vi "new_nerualnetwork_test.vi"() -> ()   [LabVIEW 2014]
panel:
  out "Output Layer":dbl[](array[numeric])
  out "HiDen Layer":dbl[](array[numeric])
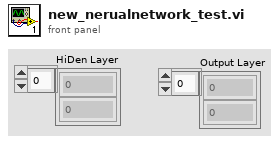
[diagram p1: front panel]
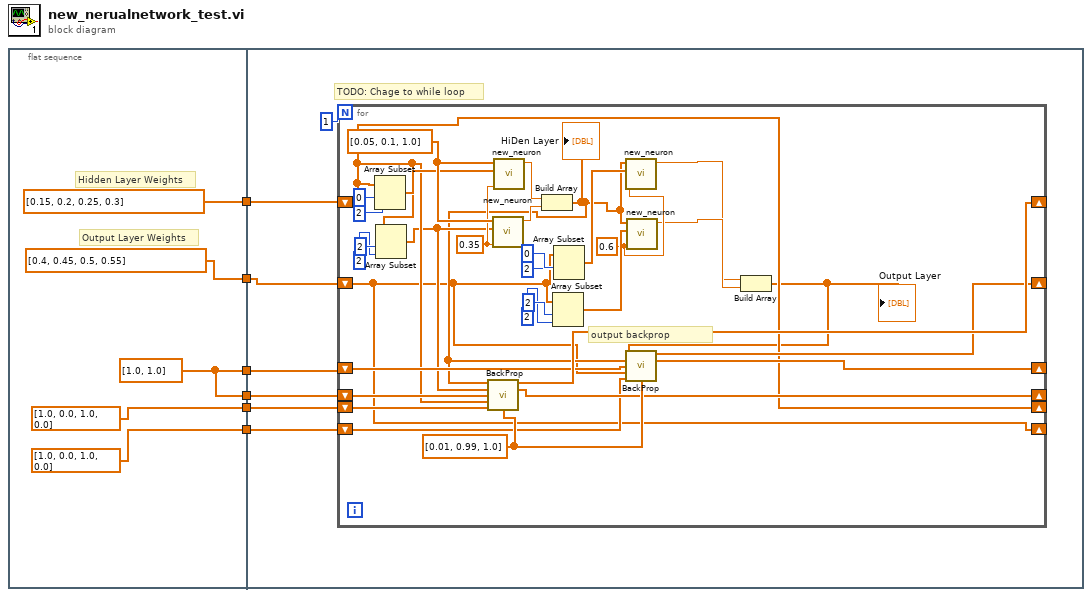
[diagram p0: block diagram]
diagram:
  n1 = flat-sequence {
    tunnel: [dbl[] [0.15, 0.2, 0.25, 0.3] ("Target")] -> w6
    tunnel: [dbl[] [0.4, 0.45, 0.5, 0.55] ("Target")] -> w5
    tunnel: [w9] -> w4
    tunnel: [w9] -> w3
    tunnel: [dbl[] [1.0, 0.0, 1.0, 0.0] ("PreviousWeights")] -> w2
    tunnel: [dbl[] [1.0, 0.0, 1.0, 0.0] ("PreviousWeights")] -> w1
    tunnel: w6 -> [w18]
    tunnel: w5 -> [w16]
    tunnel: w4 -> [w15]
    tunnel: w3 -> [w14]
    tunnel: w2 -> [w13]
    tunnel: w1 -> [w12]
    frame #0 {
      w9 = dbl[] [1.0, 1.0] ("dE_dNET")
      # "Output Layer Weights"
      # "Hidden Layer Weights"
    }
    frame #1 {
      # "TODO: Chage to while loop"
      n2 = for {
        N: 1 -> [_]
        shift-right: [w29] -> _
        shift-left: w16 -> [w19]
        shift-right: [w30] -> _
        shift-left: w18 -> [w24]
        shift-right: [w31] -> _
        shift-left: w15 -> [w26]
        shift-right: [w28] -> _
        shift-left: w14 -> [w27]
        shift-right: [w24] -> _
        shift-left: w13 -> [w25]
        shift-right: [w19] -> _
        shift-left: w12 -> [w23]
        w35 = 0.6 ("Offset")
        w36 = 0.35 ("Offset")
        w50 = dbl[] [0.05, 0.1, 1.0] ("Target")
        w32 = dbl[] [0.01, 0.99, 1.0] ("Target")
        # "output backprop"
        n3 = Array Subset(array=w24, index=0, length=2) -> (w45:dbl[])
        n4 = Array Subset(array=w24, index=2, length=2) -> (w22:dbl[])
        n5 = call "new_neuron.vi"("Offset"=w36, "Weights"=w22, "Inputs"=w50) -> ("Output"=w43:dbl)  [unwired: 8 in]
        n6 = call "new_neuron.vi"("Offset"=w36, "Weights"=w45, "Inputs"=w50) -> ("Output"=w44:dbl)  [unwired: 8 in]
        n7 = Build Array(w44, w43) -> (w21:dbl[])
        "HiDen Layer" <- w21
        n8 = call "BackProp.vi"("Current Layer"=w21, "Previous Layer"=w22, "NetError"=w27, "weights"=w24, "PreviousWeights"=w25, "Target"=w32) -> ("w+"=w30:dbl[], "dE_dNET"=w28:dbl[])  [unwired: 8 in]
        n9 = Array Subset(array=w19, index=2, length=2) -> (w38:dbl[])
        n10 = Array Subset(array=w19, index=0, length=2) -> (w37:dbl[])
        n11 = call "new_neuron.vi"("Offset"=w35, "Weights"=w37, "Inputs"=w21) -> ("Output"=w33:dbl)  [unwired: 8 in]
        n12 = call "new_neuron.vi"("Offset"=w35, "Weights"=w38, "Inputs"=w21) -> ("Output"=w34:dbl)  [unwired: 8 in]
        n13 = Build Array(w33, w34) -> (w20:dbl[])
        "Output Layer" <- w20
        n14 = call "BackProp.vi"("Current Layer"=w20, "Previous Layer"=w21, "NetError"=w26, "weights"=w19, "PreviousWeights"=w23, "Target"=w32) -> ("w+"=w29:dbl[], "dE_dNET"=w31:dbl[])  [unwired: 8 in]
      }
    }
  }
